vi "Send and receive test.vi"() -> ()   [LabVIEW 2012]
panel:
  out "byte array":u8[](array[numeric]) format="%02x"
  out "String Received":string
  out "return count":u32
  out "bytes written":u32
  out "Blinky":bool
  in  "String":string="1234"
  in  "stop":bool
  in  "VISA resource name":refnum<visa-resource-name>="COM6"
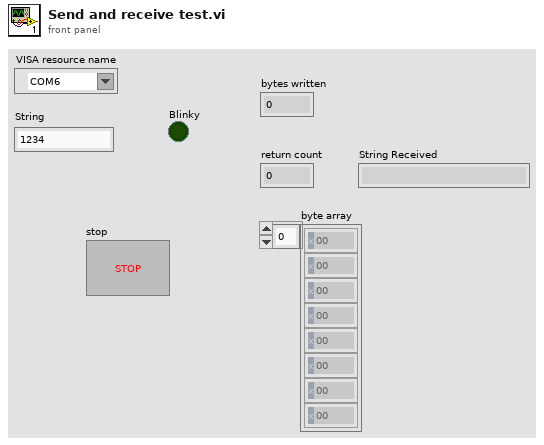
[diagram p1: front panel]
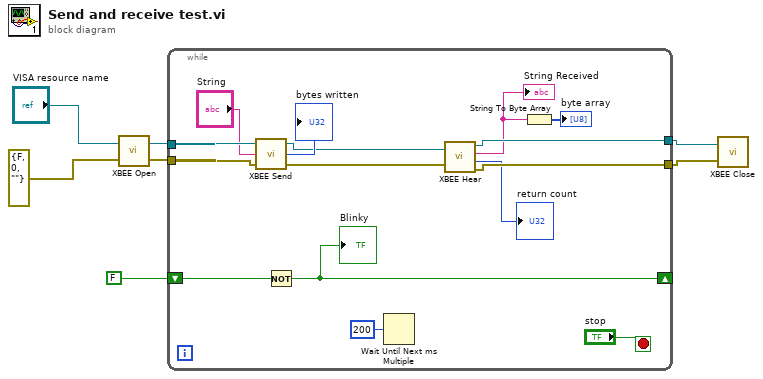
[diagram p0: block diagram]
diagram:
  n1 = call "XBEE Open.vi"("error in"=errorcluster {"status"=FALSE, "code"=0, "source"=""}, "VISA resource name"="VISA resource name") -> ("error out"=w4:errorcluster, "VISA resource name out"=w5:refnum<visa-resource-name>)
  n2 = while {
    tunnel: w5 -> [w20]
    tunnel: w4 -> [w19]
    tunnel: [w12] -> w3
    tunnel: [w11] -> w2
    shift-right: [w17] -> _
    shift-left: FALSE -> [w18]
    stop <- "stop" stop-if-true
    n3 = call "XBEE Send.vi"("error in (no error)"=w19, "String"="String", "VISA resource name"=w20) -> ("error out"=w14:errorcluster, "return count"=→"bytes written":u32, "VISA resource name out"=w13:refnum<visa-resource-name>)
    n4 = Not(x=w18) -> (.not. x?=w17:bool)
    "Blinky" <- w17
    n5 = Wait Until Next ms Multiple(millisecond multiple=u32 200) -> ()  [unwired: 1 out]
    n6 = call "XBEE Hear.vi"("VISA resource name"=w13, "error in (no error)"=w14) -> ("VISA resource name out"=w12:refnum<visa-resource-name>, "String Received"=w9:string, "return count"=→"return count":u32, "error out"=w11:errorcluster)
    "String Received" <- w9
    n7 = String To Byte Array(string=w9) -> (unsigned byte array=→"byte array":u8[])
  }
  n8 = call "XBEE Close.vi"("error in (no error)"=w2, "VISA resource name"=w3) -> ()
